vi "VIP_Post-Uninstall Custom Action.vi"(10 "Variant":variant) -> (0 "error out":errorcluster)   [LabVIEW 2021]
uses:
  <vilib>/zip/NI_Unzip.lvlib
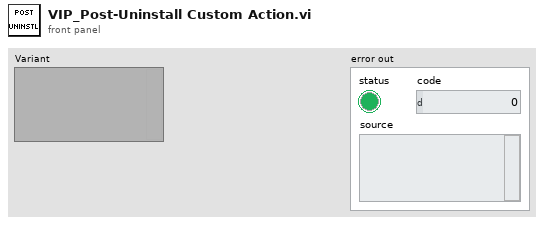
[diagram p1: front panel]
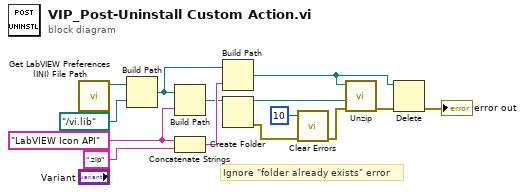
[diagram p0: block diagram]
diagram:
  w6 = "LabVIEW Icon API"
  # "Ignore \"folder already exists\" error"
  n1 = call <resource>:"Get LabVIEW Preferences (INI) File Path.vi"() -> ("LabVIEW Preferences (INI) File Path"=w8:path)  [unwired: 11 in]
  n2 = Build Path(base path=w8, name or relative path=path "../vi.lib" ("symbolic path")) -> (appended path=w4:path)
  n3 = Build Path(base path=w4, name or relative path=w6) -> (appended path=w1:path)
  n4 = Concatenate Strings(w6, ".zip" ("string")) -> (w3:string)
  n5 = Build Path(base path=w4, name or relative path=w3) -> (appended path=w2:path)
  n6 = Create Folder(path (use dialog)=w1) -> (created path=w10:path, error out=w14:errorcluster)  [unwired: 2 in, 1 out]
  n7 = call <vilib>:"Clear Errors.vi"("error in (no error)"=w14, "specific error code to clear (0: all)"=10) -> ("error out"=w13:errorcluster)  [unwired: 4 in, 1 out]
  n8 = call <vilib>:"Unzip.vi"("error in (no error)"=w13, "Target directory (same as Zip file if empty)"=w10, "Zip file"=w2) -> ("error out"=w12:errorcluster)  [unwired: 6 in, 2 out]
  n9 = Delete(path (use dialog)=w2, error in=w12) -> (error out=→"error out":errorcluster)  [unwired: 3 in, 2 out]
